vi "String_Breaker_SubVi.vi"(8 "string":string="FPSP0RP0FS0TL0PP50%TD1000FEBL1CL0RL1FL0AL1HL1G3") -> (10 "AL - 0":string, 12 "HL":string, 14 "Gear":string, 15 "BL - 0":string, 16 "FP":string, 17 "FE":string, 18 "SP - 0000":string, 19 "TD - 0000":string, 20 "FL - 0":string, 21 "RP - 0000":string, 22 "RL - 0":string, 23 "FS - 0000":string, 24 "CL - 0":string, 25 "TL - 0000":string, 26 "PP - 0000":string)   [LabVIEW 2014]
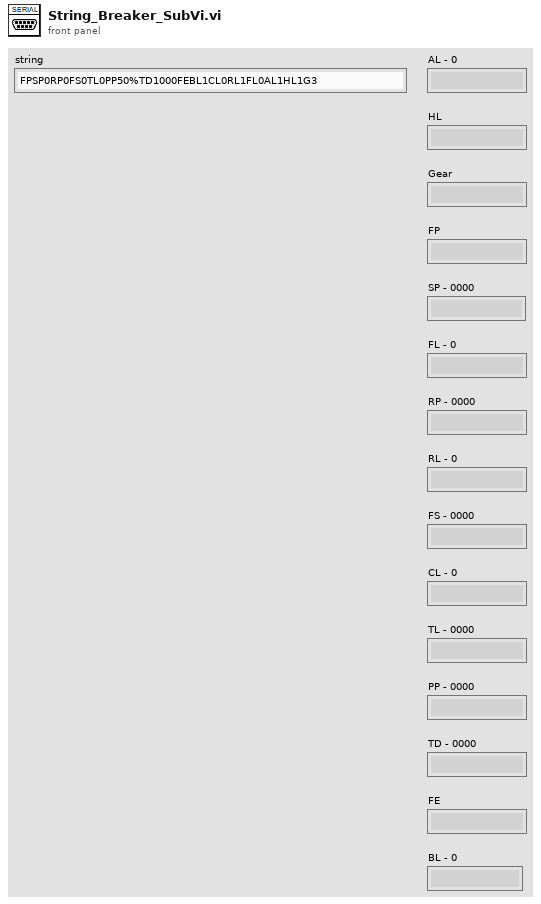
[diagram p1: front panel]
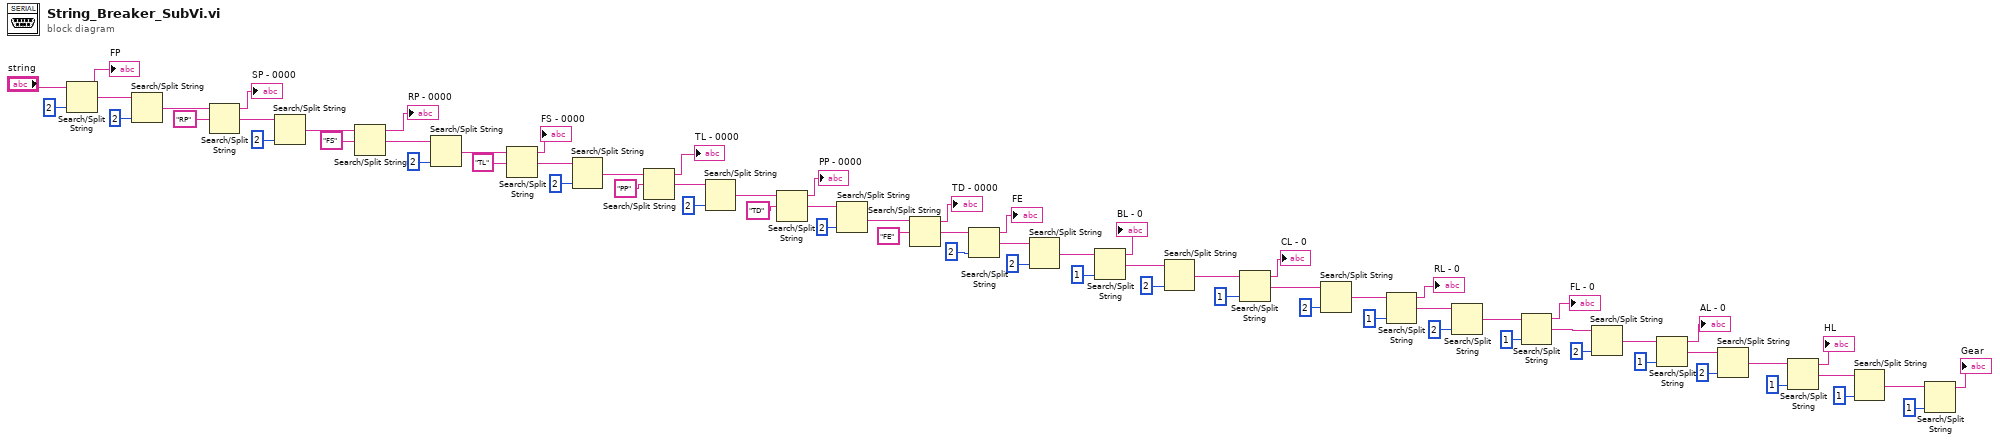
[diagram p0: block diagram]
diagram:
  n1 = Search/Split String(string="string", offset (0)=2) -> (substring before match=→"FP":string, match + rest of string=w17:string)  [unwired: 1 in, 1 out]
  n2 = Search/Split String(string=w17, offset (0)=2) -> (match + rest of string=w29:string)  [unwired: 1 in, 2 out]
  n3 = Search/Split String(string=w29, search string/char (-)="RP") -> (substring before match=→"SP - 0000":string, match + rest of string=w27:string)  [unwired: 1 in, 1 out]
  n4 = Search/Split String(string=w27, offset (0)=2) -> (match + rest of string=w25:string)  [unwired: 1 in, 2 out]
  n5 = Search/Split String(string=w25, search string/char (-)="FS") -> (substring before match=→"RP - 0000":string, match + rest of string=w24:string)  [unwired: 1 in, 1 out]
  n6 = Search/Split String(string=w24, offset (0)=2) -> (match + rest of string=w22:string)  [unwired: 1 in, 2 out]
  n7 = Search/Split String(string=w22, search string/char (-)="TL") -> (substring before match=→"FS - 0000":string, match + rest of string=w19:string)  [unwired: 1 in, 1 out]
  n8 = Search/Split String(string=w19, offset (0)=2) -> (match + rest of string=w62:string)  [unwired: 1 in, 2 out]
  n9 = Search/Split String(string=w62, search string/char (-)="PP") -> (substring before match=→"TL - 0000":string, match + rest of string=w68:string)  [unwired: 1 in, 1 out]
  n10 = Search/Split String(string=w68, offset (0)=2) -> (match + rest of string=w63:string)  [unwired: 1 in, 2 out]
  n11 = Search/Split String(string=w63, search string/char (-)="TD") -> (substring before match=→"PP - 0000":string, match + rest of string=w70:string)  [unwired: 1 in, 1 out]
  n12 = Search/Split String(string=w70, offset (0)=2) -> (match + rest of string=w71:string)  [unwired: 1 in, 2 out]
  n13 = Search/Split String(string=w71, search string/char (-)="FE") -> (substring before match=→"TD - 0000":string, match + rest of string=w42:string)  [unwired: 1 in, 1 out]
  n14 = Search/Split String(string=w42, offset (0)=2) -> (substring before match=→"FE":string, match + rest of string=w45:string)  [unwired: 1 in, 1 out]
  n15 = Search/Split String(string=w45, offset (0)=2) -> (match + rest of string=w38:string)  [unwired: 1 in, 2 out]
  n16 = Search/Split String(string=w38, offset (0)=1) -> (substring before match=→"BL - 0":string, match + rest of string=w47:string)  [unwired: 1 in, 1 out]
  n17 = Search/Split String(string=w47, offset (0)=2) -> (match + rest of string=w41:string)  [unwired: 1 in, 2 out]
  n18 = Search/Split String(string=w41, offset (0)=1) -> (substring before match=→"CL - 0":string, match + rest of string=w44:string)  [unwired: 1 in, 1 out]
  n19 = Search/Split String(string=w44, offset (0)=2) -> (match + rest of string=w50:string)  [unwired: 1 in, 2 out]
  n20 = Search/Split String(string=w50, offset (0)=1) -> (substring before match=→"RL - 0":string, match + rest of string=w53:string)  [unwired: 1 in, 1 out]
  n21 = Search/Split String(string=w53, offset (0)=2) -> (match + rest of string=w11:string)  [unwired: 1 in, 2 out]
  n22 = Search/Split String(string=w11, offset (0)=1) -> (substring before match=→"FL - 0":string, match + rest of string=w8:string)  [unwired: 1 in, 1 out]
  n23 = Search/Split String(string=w8, offset (0)=2) -> (match + rest of string=w14:string)  [unwired: 1 in, 2 out]
  n24 = Search/Split String(string=w14, offset (0)=1) -> (substring before match=→"AL - 0":string, match + rest of string=w56:string)  [unwired: 1 in, 1 out]
  n25 = Search/Split String(string=w56, offset (0)=2) -> (match + rest of string=w58:string)  [unwired: 1 in, 2 out]
  n26 = Search/Split String(string=w58, offset (0)=1) -> (substring before match=→"HL":string, match + rest of string=w1:string)  [unwired: 1 in, 1 out]
  n27 = Search/Split String(string=w1, offset (0)=1) -> (match + rest of string=w4:string)  [unwired: 1 in, 2 out]
  n28 = Search/Split String(string=w4, offset (0)=1) -> (substring before match=→"Gear":string)  [unwired: 1 in, 2 out]
